vi "pathplan_write.vi"(7 "VISA资源名称":refnum<visa-resource-name>, 8 "angle":dbl[](array[numeric]), 9 "v":dbl[](array[numeric]), 10 "y":dbl[](array[numeric]), 11 "angle_err":dbl[](array[numeric])) -> (2 "路径规划数据写入缓冲区":string)   [LabVIEW 2016]
uses:
  <vilib>/Instr/_visa.llb/VISA Configure Serial Port (Instr).vi
panel:
  out "错误输出":errorcluster
  in  "串口配置":T1={"波特率"=115200, "奇偶校验位"=0, "停止位"=10, "流控制"=0, "数据位"=8} {"数据位" items=["8"=8]; "流控制" items=["无"=0, "XON/XOFF"=1, "RTS/CTS"=2, "DTR/DSR"=4]; "停止位" items=["1.0"=10, "2.0"=15, "3.0"=20]; "奇偶校验位" items=["None"]; "波特率" items=["115200"=115200]}
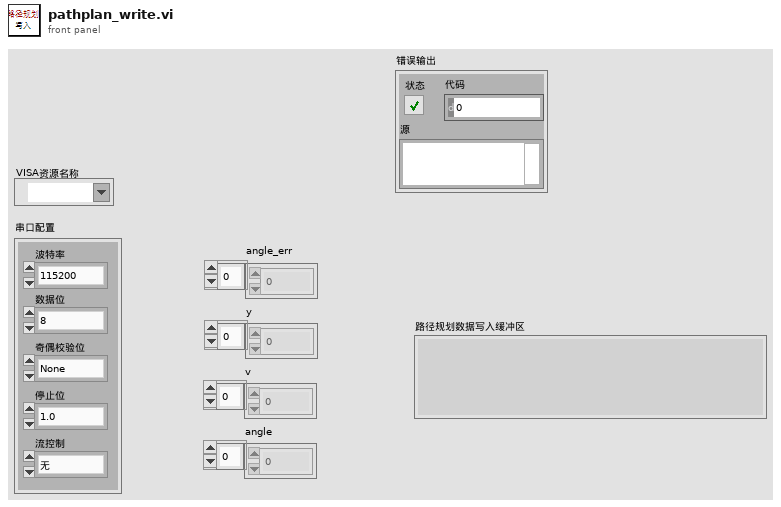
[diagram p1: front panel]
types:
  T1 = cluster{"波特率":u32, "奇偶校验位":u16, "停止位":u16, "流控制":u16, "数据位":u32}
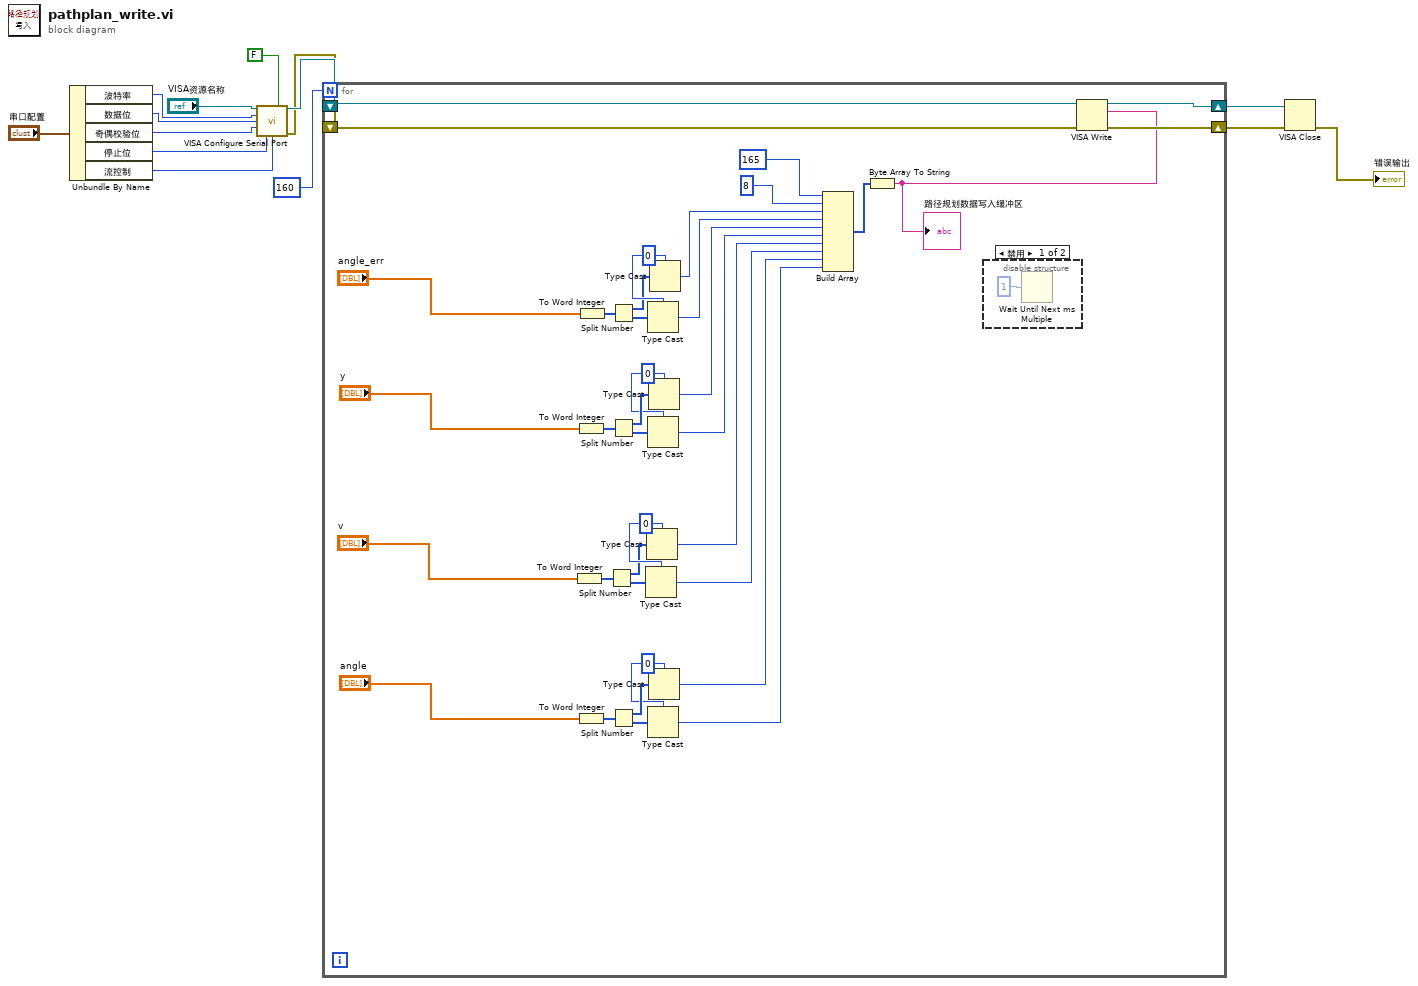
[diagram p0: block diagram]
diagram:
  n1 = Unbundle By Name("串口配置") -> ("波特率"=w12:u32, "数据位"=w11:u32, "奇偶校验位"=w10:u16, "停止位"=w9:u16, "流控制"=w8:u16)
  n2 = call-poly "VISA Configure Serial Port"("VISA resource name"="VISA资源名称", "Enable Termination\nChar (T)"=FALSE ("Enable Termination\nChar (T)"), "baud rate (9600)"=w12, "data bits (8)"=w11, "parity (0:none)"=w10, "stop bits (10: 1 bit)"=w9, "flow control (0:none)"=w8) -> ("VISA resource name out"=w5:refnum<visa-resource-name>, "error out"=w4:errorcluster)  [unwired: 7 in]
  n3 = for {
    N: 160 -> [_]
    shift-right: [w48] -> w3
    shift-left: w5 -> [w50]
    shift-right: [w47] -> w2
    shift-left: w4 -> [w49]
    w22 = u8 0
    w31 = u8 0
    w36 = u8 0
    w42 = u8 0
    n4 = To Word Integer(number="v") -> (16bit integer=w30:i16[])
    n5 = To Word Integer(number="y") -> (16bit integer=w37:i16[])
    n6 = To Word Integer(number="angle") -> (16bit integer=w23:i16[])
    n7 = To Word Integer(number="angle_err") -> (16bit integer=w40:i16[])
    n8 = Split Number(x=w30) -> (hi(x)=w29:u8[], lo(x)=w28:u8[])
    n9 = Split Number(x=w40) -> (hi(x)=w41:u8[], lo(x)=w43:u8[])
    n10 = Split Number(x=w37) -> (hi(x)=w38:u8[], lo(x)=w39:u8[])
    n11 = Split Number(x=w23) -> (hi(x)=w24:u8[], lo(x)=w25:u8[])
    n12 = Type Cast(type=w31, x=w28) -> (*(type *) &x=w18:u8)
    n13 = Type Cast(type=w31, x=w29) -> (*(type *) &x=w19:u8)
    n14 = Type Cast(type=w42, x=w43) -> (*(type *) &x=w32:u8)
    n15 = Type Cast(type=w36, x=w39) -> (*(type *) &x=w20:u8)
    n16 = Type Cast(type=w22, x=w25) -> (*(type *) &x=w16:u8)
    n17 = Type Cast(type=w36, x=w38) -> (*(type *) &x=w21:u8)
    n18 = Type Cast(type=w22, x=w24) -> (*(type *) &x=w17:u8)
    n19 = Type Cast(type=w42, x=w41) -> (*(type *) &x=w33:u8)
    n20 = Build Array(u8 165, u8 8, w33, w32, w21, w20, w19, w18, w17, w16) -> (w15:u8[])
    n21 = Byte Array To String(unsigned byte array=w15) -> (string=w46:string)
    "路径规划数据写入缓冲区" <- w46
    n22 = disable-structure shown="禁用" {
      frame Disabled {
        n23 = Wait Until Next ms Multiple(millisecond multiple=u32 1 ("毫秒倍数")) -> ()  [unwired: 1 out]
      }
      frame Enabled {
      }
    }
    n24 = VISA Write(VISA resource name=w50, write buffer=w46, error in (no error)=w49) -> (VISA resource name out=w48:refnum<visa-resource-name>, error out=w47:errorcluster)  [unwired: 1 out]
  }
  n25 = VISA Close(VISA resource name=w3, error in (no error)=w2) -> (error out=→"错误输出":errorcluster)
